vi "time_dependent_measurement.vi"() -> ()   [LabVIEW 2011]
uses:
  <vilib>/Utility/file.llb/Write To Spreadsheet File (DBL).vi
  <vilib>/Analysis/NI_AALBase.lvlib
panel:
  out "Temp":dbl format="%0.2f"
  out "no field measurement":i32(slide) scale=0.0..100.0
  out "Degauss in Process":bool
  in  "iIndex 2":u32
  out "Waveform Chart":T1(graph)={"median"=202.95542358398438, "median"=-6.883494384765625, "median"=31.491379310344826}
  in  "?":bool
  in  "z":dbl=0.087
  in  "x":dbl=0.12
  in  "y":dbl=0.315
  in  "VISA-Ressourcenname":refnum<visa-resource-name>="COM7"
  in  "phi":dbl
  in  "theta (xy-ebene)":dbl
  in  "Magnitude (mT)":dbl=200.0
  out "DeviceID":u8=53 format="%02x"
  out "Z_Range":dbl=266.0
  out "X_Y_Range":dbl=266.0
  in  "iIndex":u32
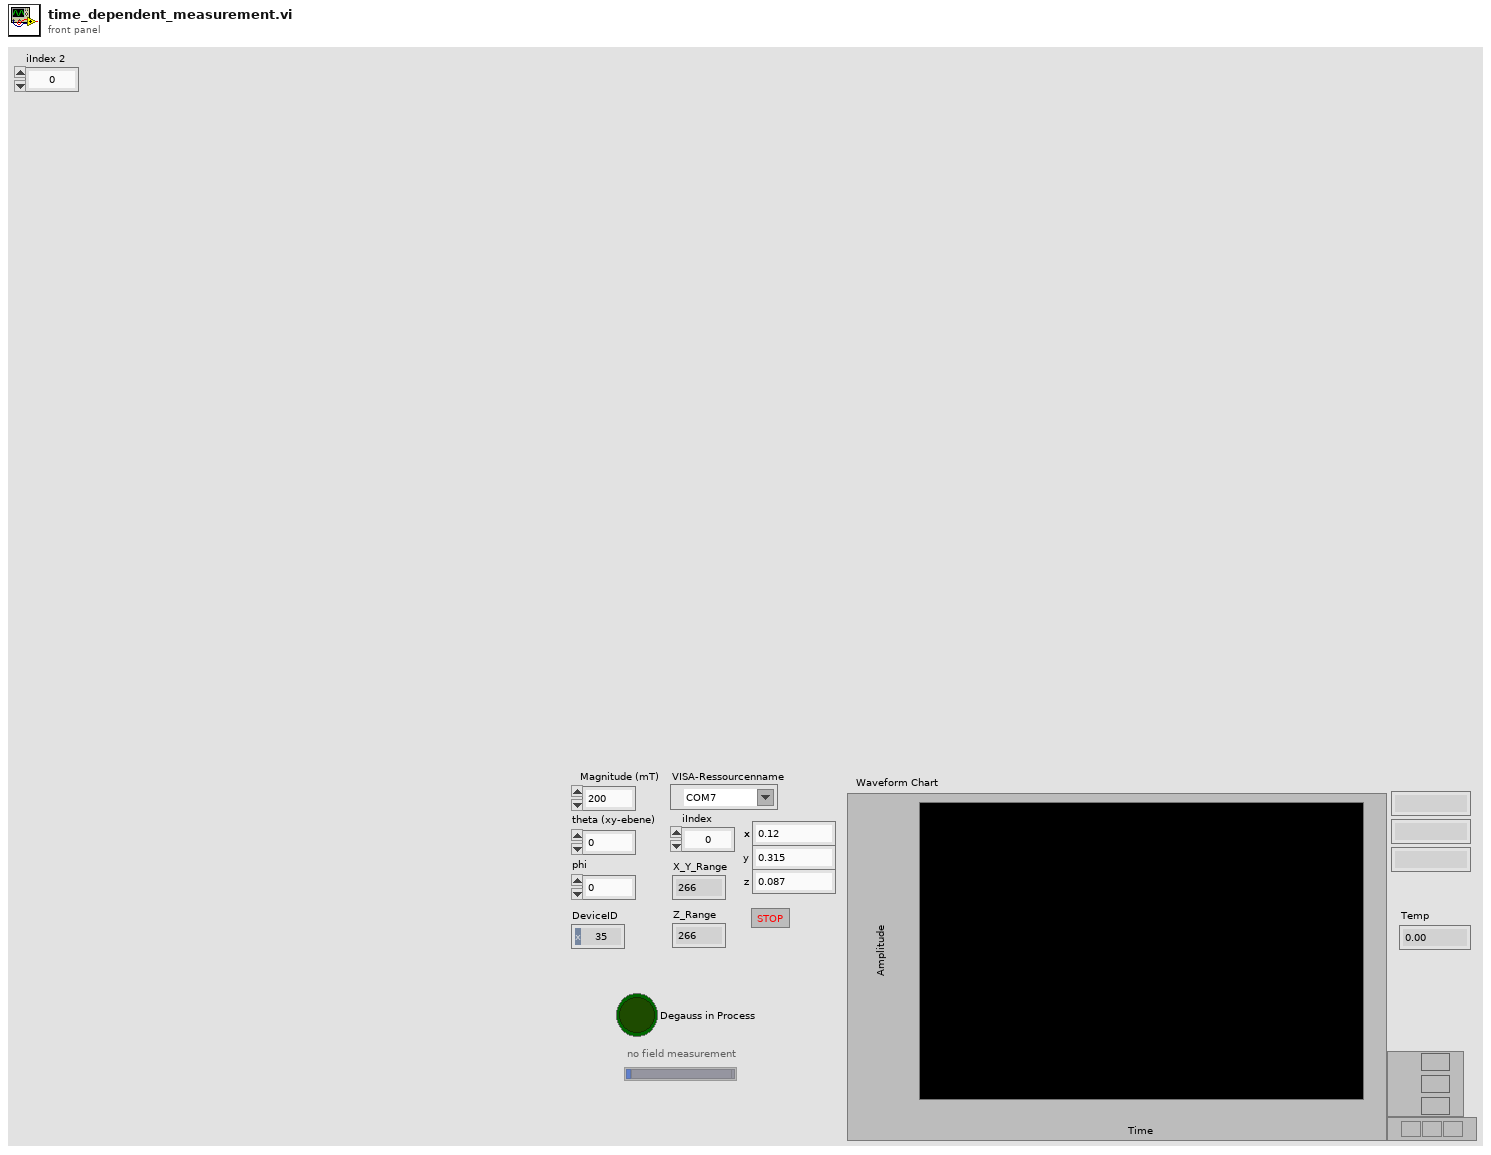
[diagram p1: front panel]
types:
  T1 = cluster{"median":dbl, "median":dbl, "median":dbl}
  T2 = enum8{"Enabled", "Disabled", "Disabled and Grayed Out"}
  T3 = enum8{"Standard I2C 3-byte read command", "1-byte I2C read command for 16bit sensor data and conversion\nstatus", "1-byte I2C read command for 8 bit sensor MSB data and\nconversion status", "Reserved"}
  T4 = cluster{"Temperature (°C)":dbl, "x (mT)":dbl, "y (mT)":dbl, "z (mT)":dbl}
  T5 = cluster{"I2C_RD":enum8{"Standard I2C 3-byte read command", "1-byte I2C read command for 16bit sensor data and conversion\nstatus", "1-byte I2C read command for 8 bit sensor MSB data and\nconversion status", "Reserved"}, "CONV_AVG":enum8{"1x average, 10.0-kSPS (3-axes) or 20-kSPS (1 axis)", "2x average, 5.7-kSPS (3-axes) or 13.3-kSPS (1 axis)", "4x average, 3.1-kSPS (3-axes) or 8.0-kSPS (1 axis)", "8x average, 1.6-kSPS (3-axes) or 4.4-kSPS (1 axis)", "16x average, 0.8-kSPS (3-axes) or 2.4-kSPS (1 axis)", "32x average, 0.4-kSPS (3-axes) or 1.2-kSPS (1 axis)"}, "MAG_TEMPCO":enum8{"0 %/°C (No temperature compensation)", "0.12 %/°C (NdBFe)", "0.03 %/°C (SmCo)", "0.20 %/°C (Ceramic)"}, "CRC_EN":enum8{"CRC disabled", "CRC enabled"}}
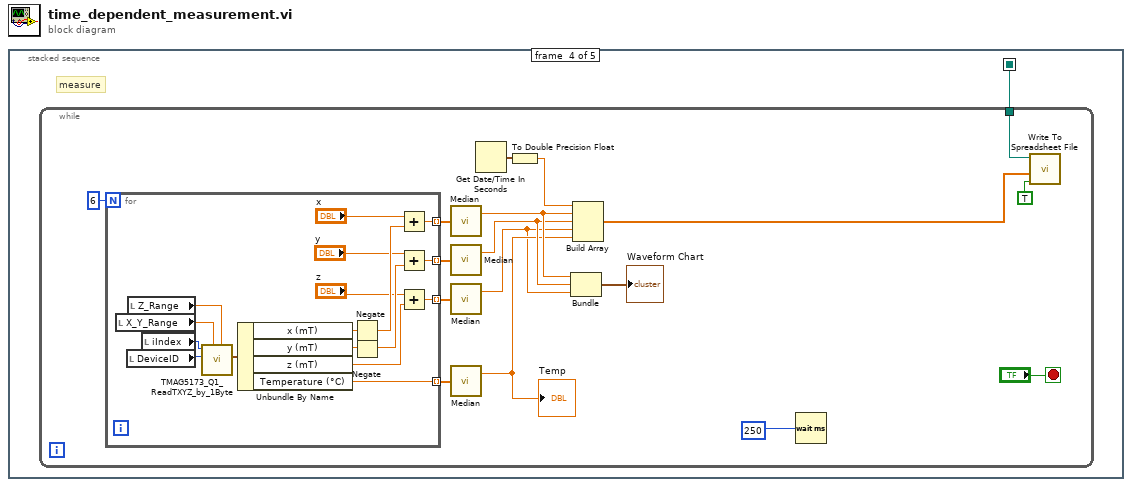
[diagram p0: block diagram]
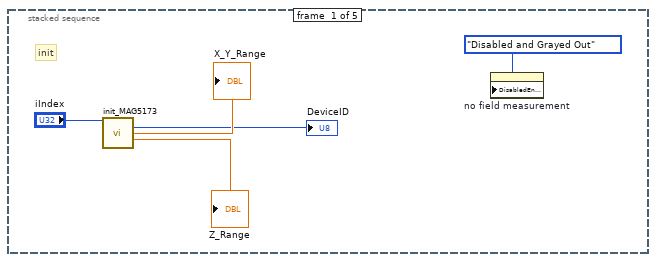
[diagram p2: hidden frame]
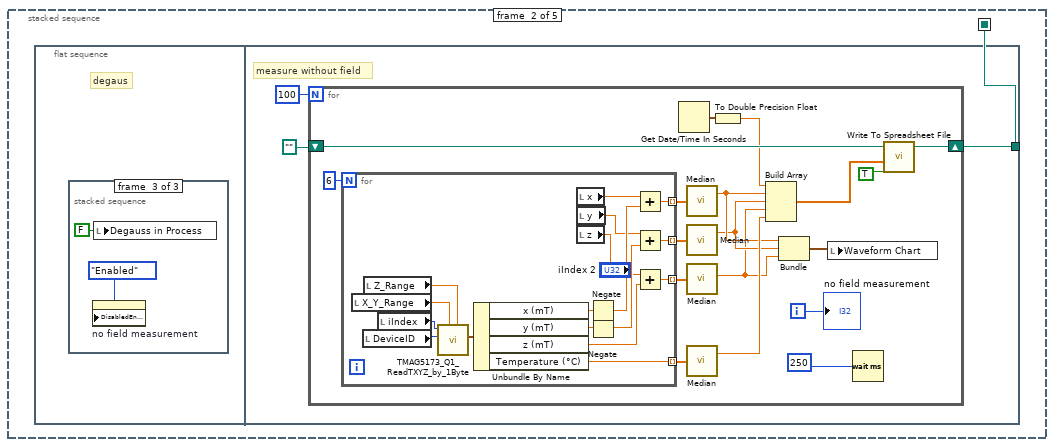
[diagram p3: hidden frame]
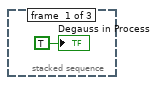
[diagram p4: hidden frame]
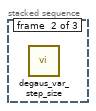
[diagram p5: hidden frame]
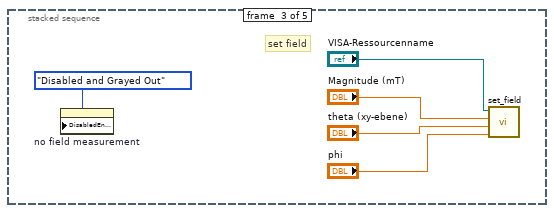
[diagram p6: hidden frame]
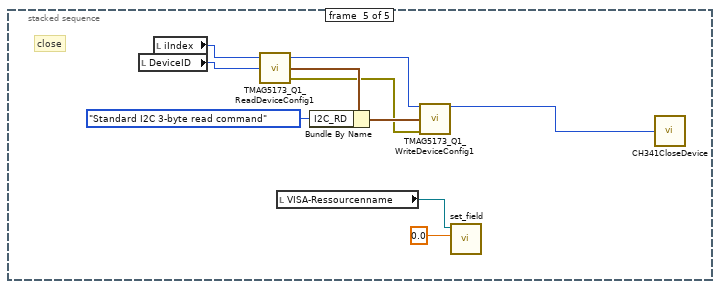
[diagram p7: hidden frame]
diagram:
  n1 = stacked-sequence {
    seq-local: [_ w6 _ _ _] -> [_ _ _ w53 _]
    frame #0 {
      # "init"
      n2 = call "init_MAG5173.vi"("iIndex"="iIndex") -> ("DeviceID"=→"DeviceID":u8, "X_Y_Range"=→"X_Y_Range":dbl, "Z_Range"=→"Z_Range":dbl)  [unwired: 10 in, 2 out]
      n3 = property on="no field measurement" class="Slide (strict)"("DisabledEnum"=T2."Disabled and Grayed Out" ("Disabled")) -> ()  [unwired: 2 in, 2 out]
    }
    frame #1 {
      n4 = flat-sequence {
        tunnel: [w11] -> w6
        frame #0 {
          # "degaus"
          n5 = stacked-sequence {
            frame #0 {
              "Degauss in Process" <- TRUE ("Degauss in Process")
            }
            frame #1 {
              n6 = call "degaus_var_step_size.vi"() -> ()  [unwired: 12 in]
            }
            frame #2 {
              n7 = property on="no field measurement" class="Slide (strict)"("DisabledEnum"=T2."Enabled" ("Disabled")) -> ()  [unwired: 2 in, 2 out]
              n8 = local write "Degauss in Process"(FALSE ("Degauss in Process")) -> ()
            }
          }
        }
        frame #1 {
          # "measure without field"
          n9 = for {
            N: 100 -> [_]
            shift-right: [w29] -> w11
            shift-left: path "" -> [w26]
            i -> [w17]
            n10 = for {
              N: 6 -> [_]
              tunnel: [w39] -> w23 mode=indexing
              tunnel: [w38] -> w22 mode=indexing
              tunnel: [w37] -> w21 mode=indexing
              tunnel: [w36] -> w24 mode=indexing
              n11 = local read "X_Y_Range"() -> (w35:dbl)
              n12 = local read "DeviceID"() -> (w46:u8)
              n13 = local read "Z_Range"() -> (w34:dbl)
              n14 = local read "iIndex"() -> (w47:u32)
              n15 = call <userlib>:"TMAG5173_Q1_ReadTXYZ_by_1Byte.vi"("z-Range"=w34, "xy-Range"=w35, "DeviceID"=w46, "iIndex"=w47) -> ("Data"=w45:T4)  [unwired: 4 in, 3 out]
              n16 = Unbundle By Name(w45) -> ("x (mT)"=w44:dbl, "y (mT)"=w43:dbl, "z (mT)"=w40:dbl, "Temperature (°C)"=w36:dbl)
              n17 = local read "x"() -> (w33:dbl)
              n18 = local read "y"() -> (w32:dbl)
              n19 = local read "z"() -> (w31:dbl)
              n20 = Negate(x=w44) -> (-x=w41:dbl)
              n21 = Negate(x=w43) -> (-x=w42:dbl)
              n22 = Add(x=w33, y=w41) -> (x+y=w39:dbl)
              n23 = Add(x=w32, y=w42) -> (x+y=w38:dbl)
              n24 = Add(x=w31, y=w40) -> (x+y=w37:dbl)
            }
            n25 = Get Date/Time In Seconds() -> (seconds since 1Jan1904=w19:timestamp)
            n26 = call <vilib>:"Median.vi"("X"=w23) -> ("median"=w16:dbl)  [unwired: 1 out]
            n27 = call <vilib>:"Median.vi"("X"=w22) -> ("median"=w15:dbl)  [unwired: 1 out]
            n28 = call <vilib>:"Median.vi"("X"=w21) -> ("median"=w14:dbl)  [unwired: 1 out]
            n29 = call <vilib>:"Median.vi"("X"=w24) -> ("median"=w20:dbl)  [unwired: 1 out]
            n30 = To Double Precision Float(number=w19) -> (double precision float=w18:dbl)
            n31 = Build Array(w18, w16, w15, w14, w20) -> (w27:dbl[])
            n32 = Bundle("median"=w16, "median"=w15, "median"=w14) -> (w13:T1)  [unwired: 1 in]
            n33 = local write "Waveform Chart"(w13) -> ()
            n34 = Wait (ms)(milliseconds to wait=u32 250) -> ()  [unwired: 1 out]
            n35 = call-poly <vilib>:"Write To Spreadsheet File.vi"("append to file? (new file:F)"=TRUE, "1D data"=w27, "file path (dialog if empty)"=w26) -> ("new file path (Not A Path if cancelled)"=w29:path)  [unwired: 5 in]
            "no field measurement" <- w17
          }
        }
      }
    }
    frame #2 {
      # "set field"
      n36 = property on="no field measurement" class="Slide (strict)"("DisabledEnum"=T2."Disabled and Grayed Out" ("Disabled")) -> ()  [unwired: 2 in, 2 out]
      n37 = call "set_field.vi"("phi"="phi", "theta (xy-ebene)"="theta (xy-ebene)", "Magnitude (mT)"="Magnitude (mT)", "VISA-Ressourcenname"="VISA-Ressourcenname") -> ()  [unwired: 8 in]
    }
    frame #3 {
      # "measure"
      n38 = while {
        tunnel: w53 -> [w63]
        stop <- "?" stop-if-true
        n39 = for {
          N: 6 -> [_]
          tunnel: [w79] -> w67 mode=indexing
          tunnel: [w78] -> w68 mode=indexing
          tunnel: [w77] -> w69 mode=indexing
          tunnel: [w76] -> w66 mode=indexing
          n40 = local read "X_Y_Range"() -> (w72:dbl)
          n41 = local read "DeviceID"() -> (w86:u8)
          n42 = local read "Z_Range"() -> (w71:dbl)
          n43 = local read "iIndex"() -> (w87:u32)
          n44 = call <userlib>:"TMAG5173_Q1_ReadTXYZ_by_1Byte.vi"("z-Range"=w71, "xy-Range"=w72, "DeviceID"=w86, "iIndex"=w87) -> ("Data"=w85:T4)  [unwired: 4 in, 3 out]
          n45 = Unbundle By Name(w85) -> ("x (mT)"=w84:dbl, "y (mT)"=w83:dbl, "z (mT)"=w80:dbl, "Temperature (°C)"=w76:dbl)
          n46 = Negate(x=w84) -> (-x=w81:dbl)
          n47 = Negate(x=w83) -> (-x=w82:dbl)
          n48 = Add(x="x", y=w81) -> (x+y=w79:dbl)
          n49 = Add(x="y", y=w82) -> (x+y=w78:dbl)
          n50 = Add(x="z", y=w80) -> (x+y=w77:dbl)
        }
        n51 = call <vilib>:"Median.vi"("X"=w67) -> ("median"=w60:dbl)  [unwired: 1 out]
        n52 = call <vilib>:"Median.vi"("X"=w68) -> ("median"=w59:dbl)  [unwired: 1 out]
        n53 = call <vilib>:"Median.vi"("X"=w69) -> ("median"=w54:dbl)  [unwired: 1 out]
        n54 = call <vilib>:"Median.vi"("X"=w66) -> ("median"=w58:dbl)  [unwired: 1 out]
        "Temp" <- w58
        n55 = Get Date/Time In Seconds() -> (seconds since 1Jan1904=w56:timestamp)
        n56 = To Double Precision Float(number=w56) -> (double precision float=w55:dbl)
        n57 = Bundle("median"=w60, "median"=w59, "median"=w54) -> (→"Waveform Chart":T1)  [unwired: 1 in]
        n58 = Build Array(w55, w60, w59, w54, w58) -> (w62:dbl[])
        n59 = Wait (ms)(milliseconds to wait=u32 250) -> ()  [unwired: 1 out]
        n60 = call-poly <vilib>:"Write To Spreadsheet File.vi"("append to file? (new file:F)"=TRUE, "1D data"=w62, "file path (dialog if empty)"=w63) -> ()  [unwired: 5 in, 1 out]
      }
    }
    frame #4 {
      # "close"
      n61 = local read "DeviceID"() -> (w91:u8)
      n62 = local read "iIndex"() -> (w92:u32)
      n63 = call <userlib>:"TMAG5173_Q1_ReadDeviceConfig1.vi"("DeviceID"=w91, "iIndex"=w92) -> ("error out"=w93:errorcluster, "Device_Config_1"=w97:T5, "oIndex"=w94:u32)  [unwired: 1 in]
      n64 = local read "VISA-Ressourcenname"() -> (w88:refnum<visa-resource-name>)
      n65 = Bundle By Name(cluster=w97, "I2C_RD"=T3."Standard I2C 3-byte read command") -> (w96:T5)
      n66 = call <userlib>:"TMAG5173_Q1_WriteDeviceConfig1.vi"("iIndex"=w94, "Device_Config_1"=w96, "error in (no error)"=w93) -> ("oIndex"=w90:u32)  [unwired: 10 in, 2 out]
      n67 = call "set_field.vi"("Magnitude (mT)"=0.0, "VISA-Ressourcenname"=w88) -> ()  [unwired: 10 in]
      n68 = call <userlib>:"CH341CloseDevice.vi"("iIndex"=w90) -> ()  [unwired: 1 in]
    }
  }
